vi "Easy_Mathematics.vi"() -> ()   [LabVIEW 2022 SP3]
panel:
  out "Multiplication":dbl
  in  "stop":bool
  out "Division":dbl
  out "Subtraction":dbl
  out "Addition":dbl
  in  "Variable 2":dbl=1.0
  in  "Variable 1":dbl=1.0
  # "Lab 1: Assignment 1"
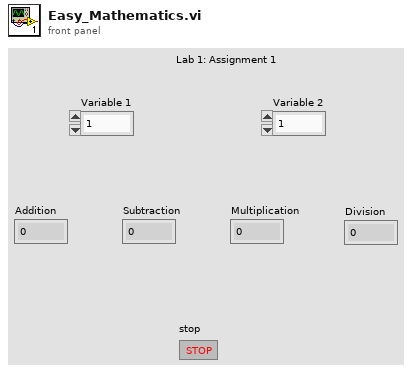
[diagram p1: front panel]
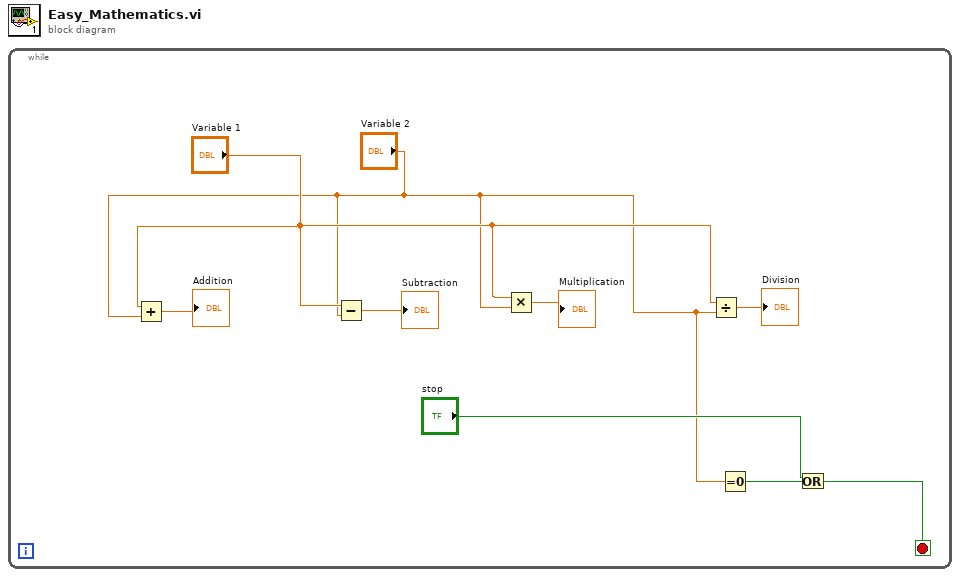
[diagram p0: block diagram]
diagram:
  n1 = while {
    stop <- w3 stop-if-true
    n2 = Add(x="Variable 1", y="Variable 2") -> (x+y=→"Addition":dbl)
    n3 = Subtract(x="Variable 1", y="Variable 2") -> (x-y=→"Subtraction":dbl)
    n4 = Multiply(x="Variable 1", y="Variable 2") -> (x*y=→"Multiplication":dbl)
    n5 = Divide(x="Variable 1", y="Variable 2") -> (x/y=→"Division":dbl)
    n6 = Equal To 0?(x="Variable 2") -> (x = 0?=w4:bool)
    n7 = Or(x="stop", y=w4) -> (x .or. y?=w3:bool)
  }
